vi "F Dwf Digital In Trigger Set.vi"(6 "fsEdgeFall":u32, 7 "fsEdgeRise":u32, 8 "error in (no error)":errorcluster, 9 "fsLevelHigh":u32, 10 "fsLevelLow":u32, 11 "hdwf":i32) -> (0 "error out":errorcluster, 3 "function return":i32)   [LabVIEW 2019, in "Olasdwf.lvlib"]
doc: "DWFAPI int FDwfDigitalInTriggerSet(HDWF hdwf, unsigned int fsLevelLow, unsigned int fsLevelHigh, unsigned int fsEdgeRise, unsigned int fsEdgeFall);"
uses:
  Olasdwf.lvlib
  Windows/System32/dwf.dll
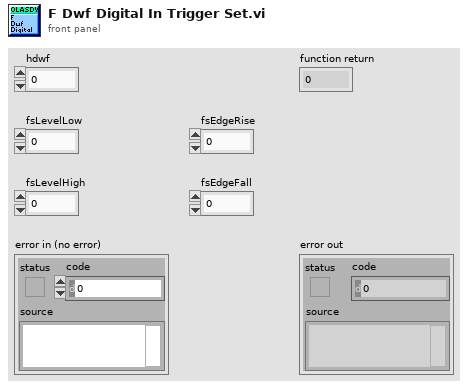
[diagram p1: front panel]
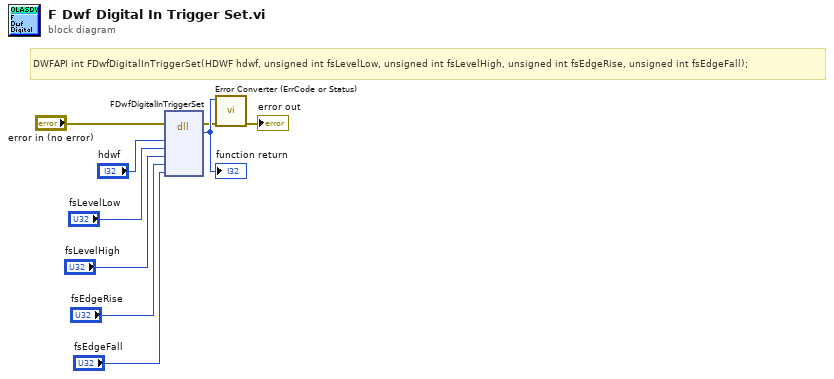
[diagram p0: block diagram]
diagram:
  # "DWFAPI int FDwfDigitalInTriggerSet(HDWF hdwf, unsigned int fsLevelLow, unsigned int fsLevelHigh, unsigned int fsEdgeRise, unsigned int fsEdgeFall);"
  n1 = dll-call lib="C:/Windows/System32/dwf.*" fn="FDwfDigitalInTriggerSet"(error in="error in (no error)", "hdwf"="hdwf", "fsLevelLow"="fsLevelLow", "fsLevelHigh"="fsLevelHigh", "fsEdgeRise"="fsEdgeRise", "fsEdgeFall"="fsEdgeFall") -> (error out=w2:errorcluster, w9:i32)  [unwired: 7 in, 1 out]
  "function return" <- w9
  n2 = call "Error Converter (ErrCode or Status).vi"("error in (no error)"=w2, "error code"=w9) -> ("error out"=→"error out":errorcluster)  [unwired: 9 in]
